vi "Execute.vi"(8 "error in (no error)":errorcluster, 9 "System in":refnum<class "System.lvclass">, 10 "Command in":refnum<class "Command.lvclass">, 11 "BL-Extending-State in":refnum<class "BL-Extending-State.lvclass">) -> (0 "error out":errorcluster, 2 "Next State":refnum<class "State.lvclass">, 3 "BL-Extending-State out":refnum<class "BL-Extending-State.lvclass">)   [LabVIEW 2013, in "BL-Extending-State.lvclass"]
uses:
  BL-Extending-State.lvclass
  Commands/Command/Command.lvclass
  Systems/System/System.lvclass
  State/State.lvclass
  Systems/Blocker/Blocker.lvclass
  Robot Global Data.vi
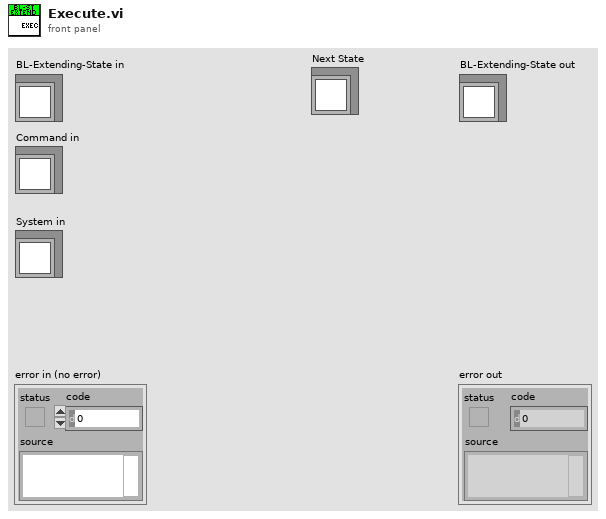
[diagram p1: front panel]
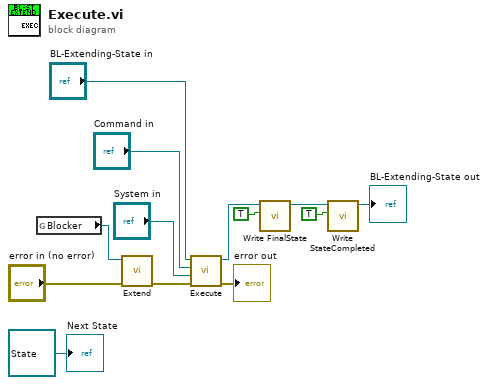
[diagram p0: block diagram]
diagram:
  n1 = global read "Robot Global Data.vi" "Blocker"() -> (w9:refnum<class "Blocker.lvclass">)
  n2 = call-dynamic "Extend.vi"("error in (no error)"="error in (no error)", "Blocker in"=w9) -> ("error out"=w7:errorcluster)  [unwired: 8 in, 1 out]
  n3 = call-parent "Execute.vi"("error in (no error)"=w7, "System in"="System in", "Command in"="Command in", "State in"="BL-Extending-State in") -> ("error out"=→"error out":errorcluster, "State out"=w4:refnum<class "BL-Extending-State.lvclass">)  [unwired: 5 in, 1 out]
  n4 = call-dynamic "Write FinalState.vi"("FinalState"=TRUE, "State in"=w4) -> ("State out"=w5:refnum<class "BL-Extending-State.lvclass">)  [unwired: 8 in, 1 out]
  n5 = call-dynamic "Write StateCompleted.vi"("StateCompleted"=TRUE, "State in"=w5) -> ("State out"=→"BL-Extending-State out":refnum<class "BL-Extending-State.lvclass">)  [unwired: 8 in, 1 out]
  "Next State" <- refnum<class "State.lvclass"> refnum ("State.lvclass")
